vi "sub_vi_saving_string_read.vi"(0 "Received data":string[](array[string]), 2 "Mean":dbl, 3 "Standard deviation":dbl, 4 "Variance":dbl, 5 "Slope":dbl, 6 "Intercept":dbl, 7 "Conversion":dbl, 10 "Gain":dbl, 11 "Converted std dev":dbl, 15 "Converted variance":dbl, 17 "Abs error":dbl, 19 "Relative error":dbl) -> (23 "Resulting string":string[](array[string]))   [LabVIEW 2016]
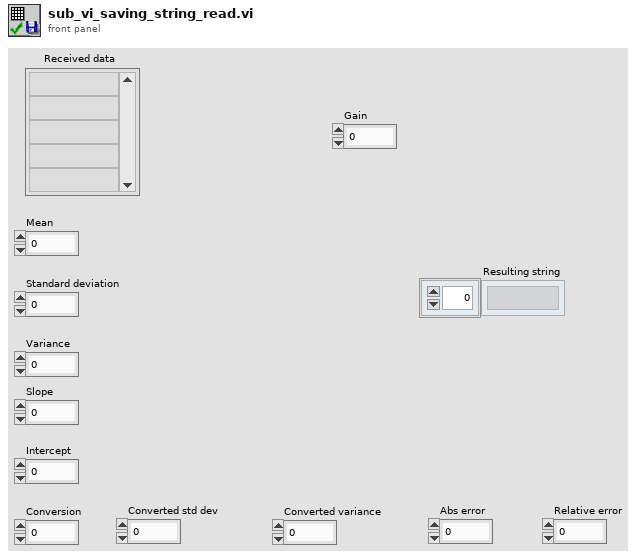
[diagram p1: front panel]
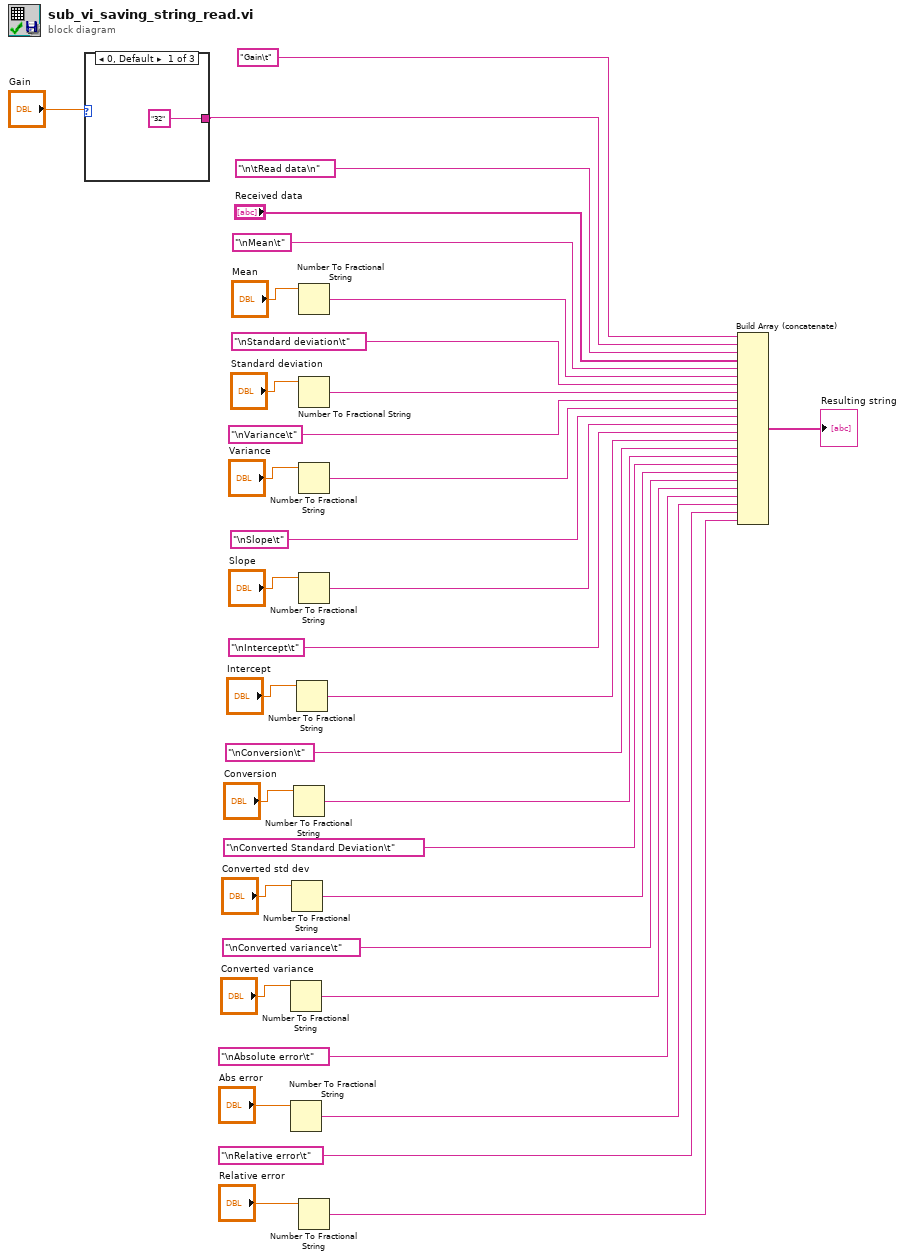
[diagram p0: block diagram]
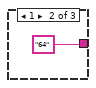
[diagram p2: hidden frame]
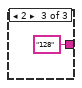
[diagram p3: hidden frame]
diagram:
  n1 = case shown="0, Default" "Gain" {
    tunnel: ["32" "64" "128"] -> w7
    frame 0, Default {
    }
    frame 1 {
    }
    frame 2 {
    }
  }
  n2 = Number To Fractional String(number="Converted variance") -> (F-format string=w10:string)  [unwired: 3 in]
  n3 = Number To Fractional String(number="Abs error") -> (F-format string=w3:string)  [unwired: 3 in]
  n4 = Number To Fractional String(number="Converted std dev") -> (F-format string=w12:string)  [unwired: 3 in]
  n5 = Number To Fractional String(number="Conversion") -> (F-format string=w17:string)  [unwired: 3 in]
  n6 = Number To Fractional String(number="Intercept") -> (F-format string=w19:string)  [unwired: 3 in]
  n7 = Number To Fractional String(number="Mean") -> (F-format string=w29:string)  [unwired: 3 in]
  n8 = Number To Fractional String(number="Standard deviation") -> (F-format string=w27:string)  [unwired: 3 in]
  n9 = Number To Fractional String(number="Variance") -> (F-format string=w25:string)  [unwired: 3 in]
  n10 = Number To Fractional String(number="Slope") -> (F-format string=w21:string)  [unwired: 3 in]
  n11 = Number To Fractional String(number="Relative error") -> (F-format string=w2:string)  [unwired: 3 in]
  n12 = Build Array (concatenate)("Gain\t", w7, "\n\tRead data\n", "Received data", "\nMean\t", w29, "\nStandard deviation\t", w27, "\nVariance\t", w25, "\nSlope\t", w21, "\nIntercept\t", w19, "\nConversion\t", w17, "\nConverted Standard Deviation\t", w12, "\nConverted variance\t", w10, "\nAbsolute error\t", w3, "\nRelative error\t", w2) -> (→"Resulting string":string[])
